vi "Convert Cluster BLOB to Bool Array.vi"(8 "error in (no error)":errorcluster, 10 "Cluster BLOB in":u8[](array[numeric])) -> (0 "error out":errorcluster, 2 "Cluster Bool Array out":bool[](array[boolean]))   [LabVIEW 2026, in "FPGA Register IO.lvlib"]
uses:
  FPGA Register IO.lvlib
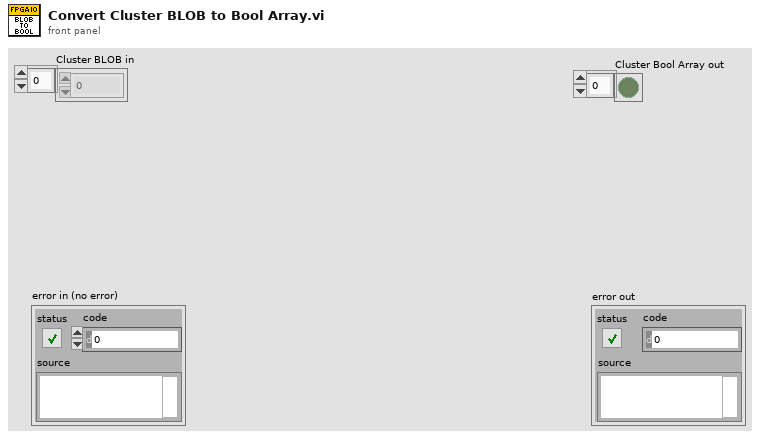
[diagram p1: front panel]
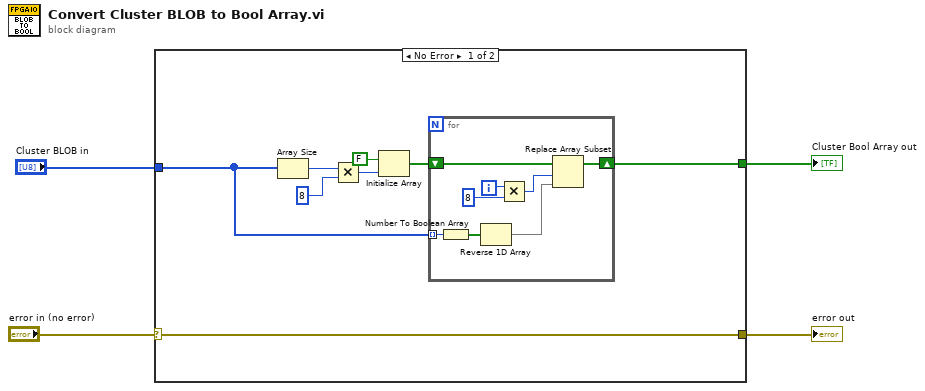
[diagram p0: block diagram]
diagram:
  n1 = case shown="No Error" "error in (no error)" {
    selector: "error in (no error)" -> [w5 w21]
    tunnel: "Cluster BLOB in" -> [w10 _]
    tunnel: [w6 _] -> w3
    tunnel: [w5 w21] -> w1
    frame No Error {
      n2 = Array Size(array=w10) -> (size(s)=w9:i32)
      n3 = Multiply(x=w9, y=8) -> (x*y=w7:i32)
      n4 = Initialize Array(FALSE, w7) -> (w11:bool[])
      n5 = for {
        tunnel: w10 -> [w20] mode=indexing
        shift-right: [w17] -> w6
        shift-left: w11 -> [w18]
        i -> [w16]
        n6 = Number To Boolean Array(number=w20) -> (Boolean array=w19:bool[])
        n7 = Reverse 1D Array(array=w19) -> (reversed array=w13:bool[])
        n8 = Multiply(x=w16, y=8) -> (x*y=w14:i32)
        n9 = Replace Array Subset(array=w18, new element=w13, index=w14) -> (w17:bool[])
      }
    }
    frame Error {
    }
  }
  "Cluster Bool Array out" <- w3
  "error out" <- w1
